vi "accuvim.vi"() -> ()   [LabVIEW 2012]
panel:
  out "Power (W)":dbl
  out "Current (A)":dbl
  out "Voltage (V)":dbl
  in  "stop":bool
  in  "Com Port of Acuvim":refnum<visa-resource-name>="COM7"
  out "frequncy (Hz)":sgl
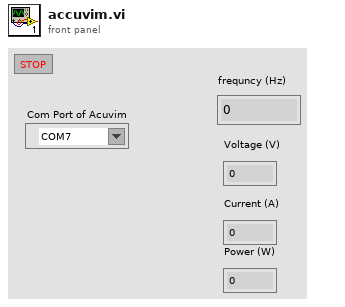
[diagram p1: front panel]
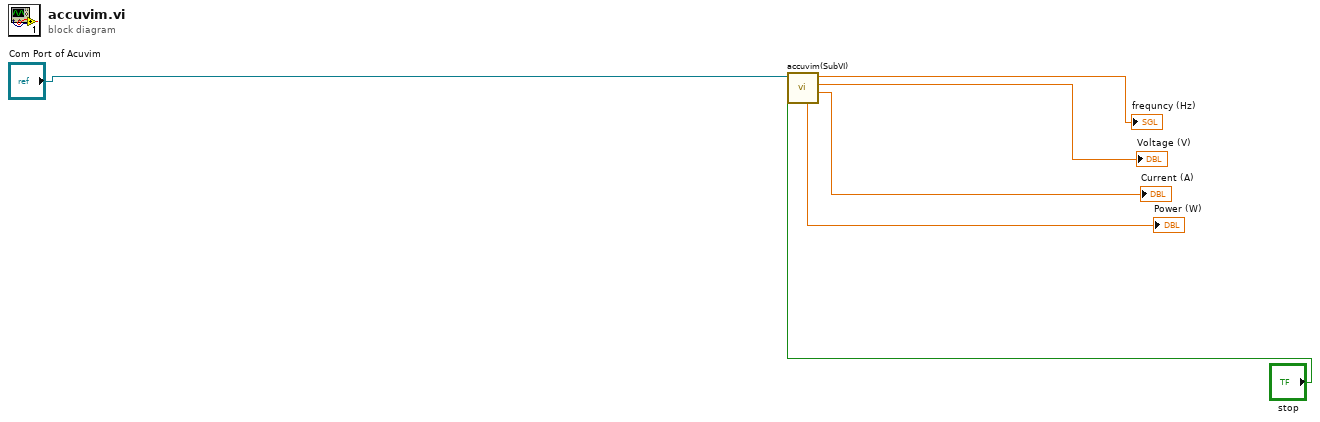
[diagram p0: block diagram]
diagram:
  n1 = call "accuvim(SubVI).vi"("stop"="stop", "VISA Refnum in"="Com Port of Acuvim") -> ("Current (A)"=→"Current (A)":dbl, "Voltage (V)"=→"Voltage (V)":dbl, "frequncy (Hz)"=→"frequncy (Hz)":sgl, "Power (W)"=→"Power (W)":dbl)  [unwired: 6 in]
